vi "Enqueue.vi"(6 "QueueArrayEntry(QMH)":T2, 7 "Enqueue Type (Enqueue)":T1=enum."Enqueue", 8 "error in (no error)":errorcluster, 9 "timeout in ms (-1)":i32, 10 "Queue Element":variant, 11 "ModuleAdmin In":refnum<class "ModuleAdmin.lvclass">) -> (0 "error out":errorcluster, 2 "MessageQueue Out":refnum<queue>, 3 "ModuleAdmin Out":refnum<class "ModuleAdmin.lvclass">)   [LabVIEW 2018, in "ModuleAdmin.lvlib" / "ModuleAdmin.lvclass"]
doc: "Enqueues an element into the queue."
uses:
  ModuleAdmin.lvclass
  TypeDefinitions/QueueEntry.ctl
  TypeDefinitions/QueueType.ctl
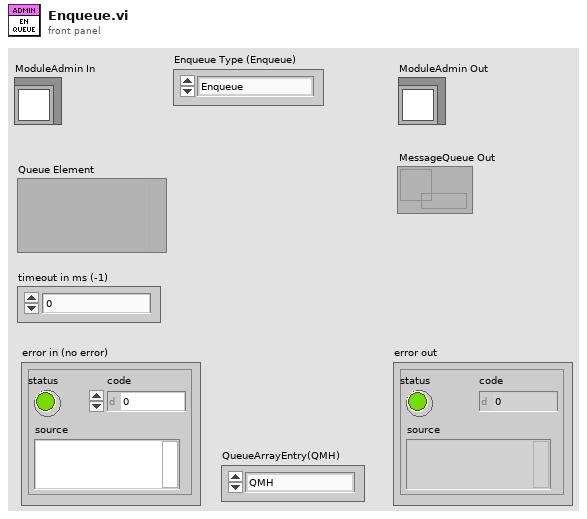
[diagram p1: front panel]
types:
  T1 = typedef "ModuleAdmin.lvlib/ModuleAdmin.lvclass/QueueType.ctl" = enum16{"EnqueueAtFront", "Enqueue", "Lossy Enqueue"}
  T2 = typedef "ModuleAdmin.lvlib/ModuleAdmin.lvclass/QueueEntry.ctl" = enum16{"QMH", "Class Data", "Data Loop", "Queue 4", "Queue 5", "Queue 6", "Queue 7", "Queue 8", "Queue 9", "Queue 10"}
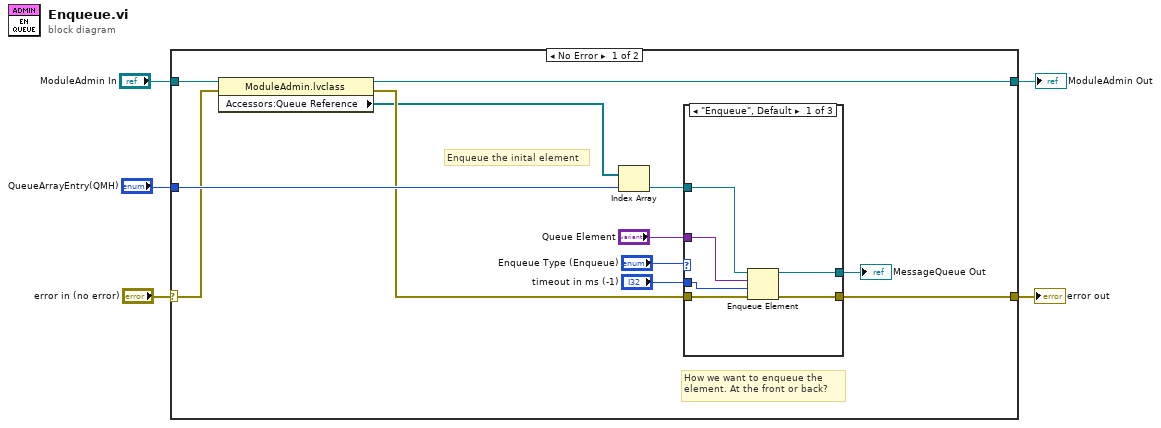
[diagram p0: block diagram]
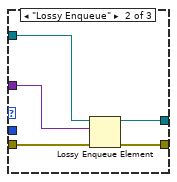
[diagram p2: hidden frame]
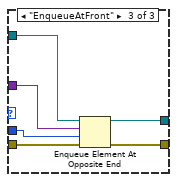
[diagram p3: hidden frame]
diagram:
  n1 = case shown="No Error" "error in (no error)" {
    selector: "error in (no error)" -> [w8 w36]
    tunnel: [w17 w36] -> w5
    tunnel: "QueueArrayEntry(QMH)" -> [w16 _]
    tunnel: "ModuleAdmin In" -> [w11 w35]
    tunnel: [w9 w35] -> w2
    frame No Error {
      # "How we want to enqueue the \nelement. At the front or back?"
      # "Enqueue the inital element"
      n2 = property class="ModuleAdmin.lvclass"(reference=w11, error in=w8) -> (reference out=w9:refnum<class "ModuleAdmin.lvclass">, error out=w7:errorcluster, "Accessors:Queue Reference"=w6:refnum<queue>[])
      n3 = Index Array(array=w6, index=w16) -> (element=w15:refnum<queue>)
      n4 = case shown="\"Enqueue\", Default" "Enqueue Type (Enqueue)" {
        tunnel: w15 -> [w23 w28 w32]
        tunnel: [w22 w26 w31] -> w13
        tunnel: [w21 w27 w33] -> w17
        tunnel: w7 -> [w20 w25 w34]
        tunnel: "timeout in ms (-1)" -> [w19 _ w30]
        tunnel: "Queue Element" -> [w18 w24 w29]
        frame "Enqueue", Default {
          n5 = Enqueue Element(queue=w23, element=w18, timeout in ms (-1)=w19, error in (no error)=w20) -> (queue out=w22:refnum<queue>, error out=w21:errorcluster)  [unwired: 1 out]
        }
        frame "Lossy Enqueue" {
          n6 = Lossy Enqueue Element(queue=w28, element=w24, error in (no error)=w25) -> (queue out=w26:refnum<queue>, error out=w27:errorcluster)  [unwired: 2 out]
        }
        frame "EnqueueAtFront" {
          n7 = Enqueue Element At Opposite End(queue=w32, element=w29, timeout in ms (-1)=w30, error in (no error)=w34) -> (queue out=w31:refnum<queue>, error out=w33:errorcluster)  [unwired: 1 out]
        }
      }
      "MessageQueue Out" <- w13
    }
    frame Error {
    }
  }
  "error out" <- w5
  "ModuleAdmin Out" <- w2
